vi "CalculatePower.vi"(6 "Reset":bool, 9 "Process Variables":cluster{"Pos":dbl, "Vel":dbl, "Accel":dbl}, 10 "Constants":T1={"FF"=0.009, "AFF"=0.002, "PID gains"={"P"=0.07, "I"=0.0, "D"=0.0}} {"PID gains"."D" format="%.3f"; "PID gains"."I" format="%.3f"; "PID gains"."P" format="%.3f"}, 11 "Setpoints":cluster{"Pos":dbl, "Vel":dbl, "Accel":dbl}) -> (3 "Power":dbl)   [LabVIEW 2016]
uses:
  <vilib>/addons/control/pid/pid.llb/PID (DBL).vi
  <vilib>/addons/control/pid/NI_PID_pid.lvlib
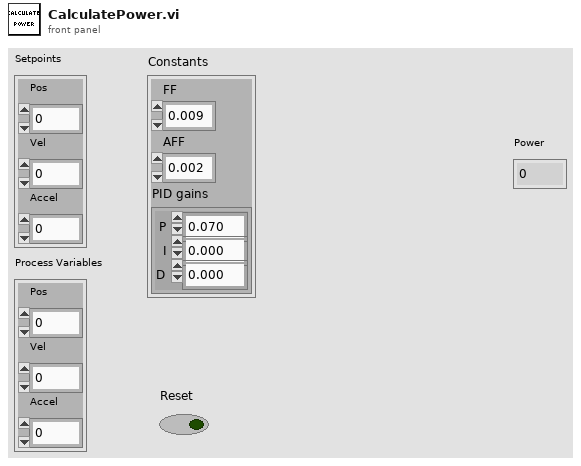
[diagram p1: front panel]
types:
  T1 = cluster{"FF":dbl, "AFF":dbl, "PID gains":cluster{"P":dbl, "I":dbl, "D":dbl}}
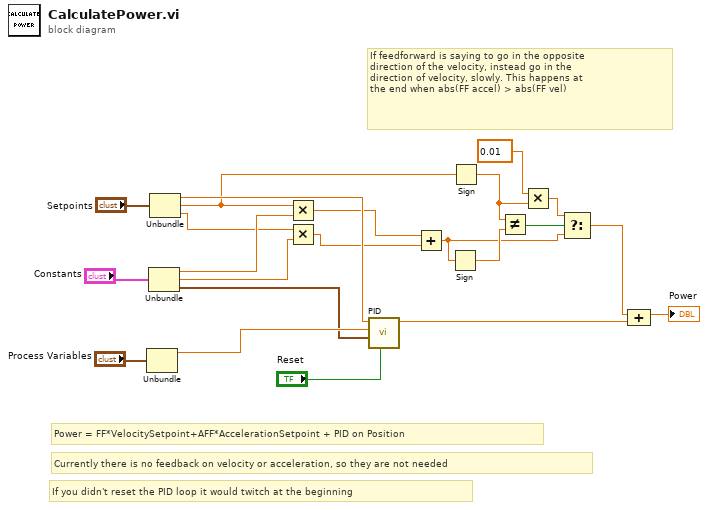
[diagram p0: block diagram]
diagram:
  # "If feedforward is saying to go in the opposite\ndirection of the velocity, instead go in the \ndirection of velocity, slowly. This happens at\nthe end when abs(FF accel) > abs(FF vel)"
  # "Currently there is no feedback on velocity or acceleration, so they are not needed"
  # "If you didn't reset the PID loop it would twitch at the beginning"
  # "Power = FF*VelocitySetpoint+AFF*AccelerationSetpoint + PID on Position"
  n1 = Unbundle("Process Variables") -> ("Pos"=w19:dbl)  [unwired: 2 out]
  n2 = Unbundle("Constants") -> ("FF"=w16:dbl, "AFF"=w15:dbl, "PID gains"=w18:cluster{"P":dbl, "I":dbl, "D":dbl})
  n3 = Unbundle("Setpoints") -> ("Pos"=w17:dbl, "Vel"=w8:dbl, "Accel"=w14:dbl)
  n4 = Multiply(x=w8, y=w16) -> (x*y=w10:dbl)
  n5 = Multiply(x=w14, y=w15) -> (x*y=w9:dbl)
  n6 = call-poly <vilib>:"PID.vi"("reinitialize? (F)"="Reset", "PID gains"=w18, "process variable"=w19, "setpoint"=w17) -> ("output"=w13:dbl)  [unwired: 6 in, 1 out]
  n7 = Add(x=w10, y=w9) -> (x+y=w5:dbl)
  n8 = Sign(1:w5) -> (0:w7:dbl)
  n9 = Sign(1:w8) -> (0:w2:dbl)
  n10 = Not Equal?(x=w2, y=w7) -> (x != y?=w6:bool)
  n11 = Multiply(x=0.01 ("t"), y=w2) -> (x*y=w4:dbl)
  n12 = Select(t=w4, s=w6, f=w5) -> (s? t:f=w1:dbl)
  n13 = Compound Arithmetic op=ADD(w1, w13) -> (→"Power":dbl)
